vi "Configure Aperture.vi"(8 "error in (no error)":errorcluster, 9 "Aperture Time (0.1 seconds)":dbl=0.1, 10 "Function (0: DC Voltage)":u16(ring) items=["DC Voltage", "AC Voltage", "2 - Wire Resistance", "4 - Wire Resistance", "DC Current", "AC Current", "Frequency", "Period", "Continuity", "Diode Checking", "VDC:VDC Ratio", "Temperature", "Capacitance"], 11 "VISA resource name":refnum<visa-resource-name>) -> (0 "error out":errorcluster, 3 "VISA resource name out":refnum<visa-resource-name>)   [LabVIEW 2020, in "Agilent 34401.lvlib"]
doc: "Configures the aperture time for applicable measurement functions.\n\n<b>Applicable Functions:</b>\n\nAll models:\n Frequency\n Period\n34410/34411 only:\n DC Voltage\n 2-Wire Resistance\n 4-Wire Resistance\n DC Current\n Temperature"
uses:
  <instrlib>/Agilent 34401/Agilent 34401.lvlib
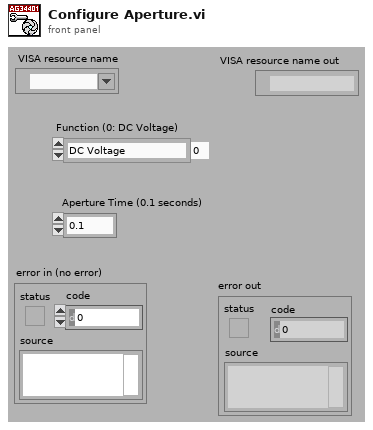
[diagram p1: front panel]
types:
  T1 = typedef "Agilent 34401.lvlib/Extended User Data.ctl" = cluster{"Trigger Source":u16, "Math Storage":u16, "Agilent Model":i32}
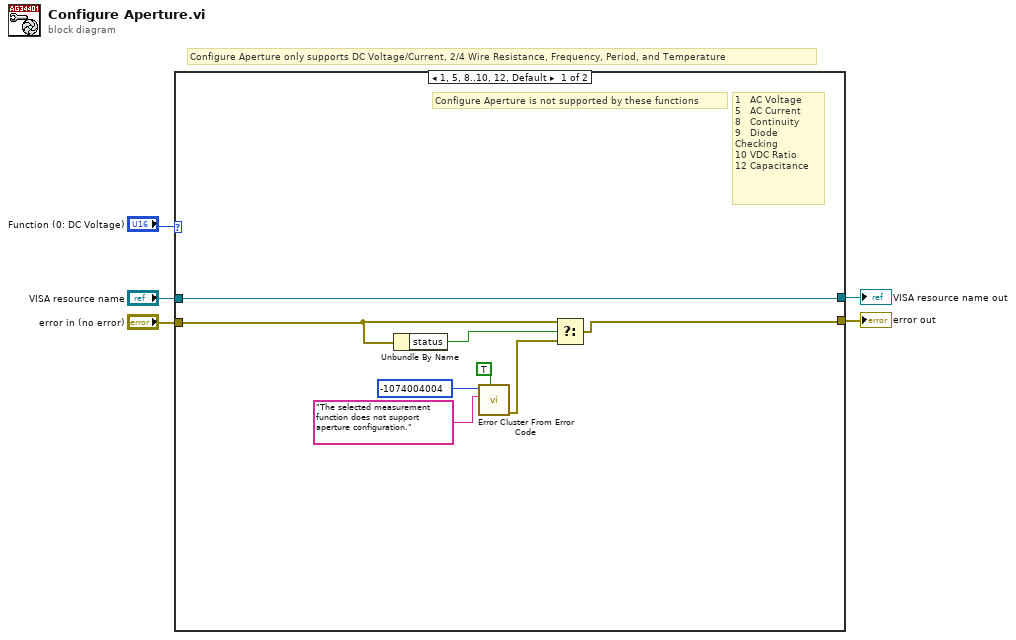
[diagram p0: block diagram]
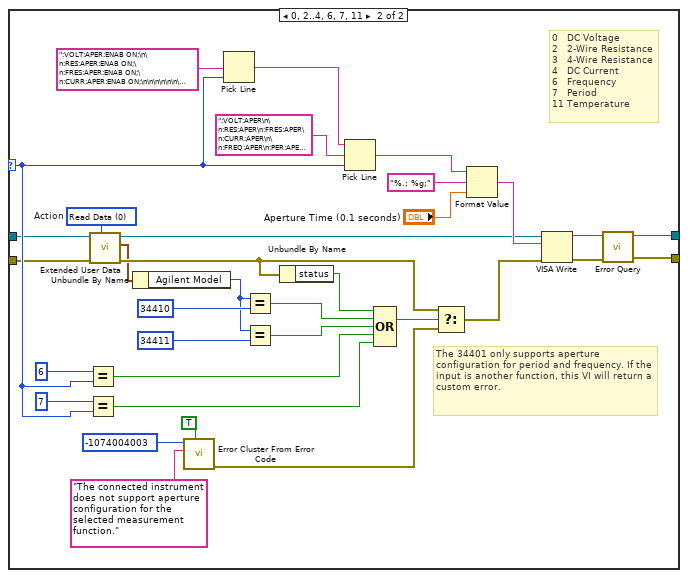
[diagram p2: hidden frame]
diagram:
  # "Configure Aperture only supports DC Voltage/Current, 2/4 Wire Resistance, Frequency, Period, and Temperature"
  n1 = case shown="1, 5, 8..10, 12, Default" "Function (0: DC Voltage)" {
    selector: "Function (0: DC Voltage)" -> [_ w34]
    tunnel: "VISA resource name" -> [w13 w20]
    tunnel: "error in (no error)" -> [w8 w19]
    tunnel: [w6 w45] -> w2
    tunnel: [w13 w44] -> w1
    frame 1, 5, 8..10, 12, Default {
      # "Configure Aperture is not supported by these functions"
      # "1   AC Voltage\n5   AC Current\n8   Continuity\n9   Diode Checking\n10 VDC Ratio \n12 Capacitance"
      n2 = Unbundle By Name(w8) -> ("status"=w9:bool)
      n3 = call <vilib>:"Error Cluster From Error Code.vi"("show call chain? (False)"=TRUE, "error message (\"\")"="The selected measurement function does not support aperture configuration." ("Source (VI Name)"), "error code (0)"=-1074004004 ("Code")) -> ("error out"=w7:errorcluster)  [unwired: 6 in]
      n4 = Select(t=w8, s=w9, f=w7) -> (s? t:f=w6:errorcluster)
    }
    frame 0, 2..4, 6, 7, 11 {
      w16 = u16 0 items=["Read Data", "Write Data", "Dispose of Data"]  # Action
      # "The 34401 only supports aperture configuration for period and frequency. If the input is another function, this VI will return a custom error."
      # "0   DC Voltage\n2   2-Wire Resistance\n3   4-Wire Resistance\n4   DC Current\n6   Frequency\n7   Period\n11 Temperature"
      n5 = Equal?(x=u16 6 ("y"), y=w34) -> (x = y?=w24:bool)
      n6 = Equal?(x=u16 7 ("y"), y=w34) -> (x = y?=w23:bool)
      n7 = call <instrlib>:"Extended User Data.vi"("Action (0: Read Data)"=w16, "Error In (no error)"=w19, "VISA resource name in"=w20) -> ("Error Out"=w17:errorcluster, "User Data Out"=w15:T1, "VISA resource name out"=w18:refnum<visa-resource-name>)  [unwired: 6 in]
      n8 = Unbundle By Name(w15) -> ("Agilent Model"=w14:i32)
      n9 = call <vilib>:"Error Cluster From Error Code.vi"("show call chain? (False)"=TRUE, "error message (\"\")"="The connected instrument does not support aperture configuration for the selected measurement function." ("Source (VI Name)"), "error code (0)"=-1074004003 ("Code")) -> ("error out"=w30:errorcluster)  [unwired: 6 in]
      n10 = Pick Line(multi-line string=":VOLT:APER:ENAB ON;\n\n:RES:APER:ENAB ON;\n:FRES:APER:ENAB ON;\n:CURR:APER:ENAB ON;\n\n\n\n\n\n\n:TEMP:APER:ENAB ON;\n", line index=w34) -> (output string=w38:string)  [unwired: 1 in]
      n11 = Equal?(x=w14, y=34410) -> (x = y?=w26:bool)
      n12 = Equal?(x=w14, y=34411) -> (x = y?=w25:bool)
      n13 = Unbundle By Name(w17) -> ("status"=w28:bool)
      n14 = Pick Line(string ("")=w38, multi-line string=":VOLT:APER\n\n:RES:APER\n:FRES:APER\n:CURR:APER\n\n:FREQ:APER\n:PER:APER\n\n\n\n:TEMP:APER\n", line index=w34) -> (output string=w21:string)
      n15 = Compound Arithmetic op=OR(w28, w26, w25, w24, w23) -> (w22:bool)
      n16 = Select(t=w17, s=w22, f=w30) -> (s? t:f=w29:errorcluster)
      n17 = Format Value(string ("")=w21, format string="%.; %g;", value (0)="Aperture Time (0.1 seconds)") -> (output string=w41:string)
      n18 = VISA Write(VISA resource name=w18, write buffer=w41, error in (no error)=w29) -> (VISA resource name out=w47:refnum<visa-resource-name>, error out=w46:errorcluster)  [unwired: 1 out]
      n19 = call <instrlib>:"Error Query.vi"("error in (no error)"=w46, "VISA resource name"=w47) -> ("error out"=w45:errorcluster, "VISA resource name out"=w44:refnum<visa-resource-name>)  [unwired: 6 in, 2 out]
    }
  }
  "error out" <- w2
  "VISA resource name out" <- w1
